vi "Read Multi Digital.vi"(0 "Device ID":T3(ring), 5 "Module":T2(array[ring]), 7 "Digital Input":T1(array[ring]), 11 "error in":errorcluster) -> (4 "Device ID Out":T3(ring), 6 "Value":bool[](array[boolean]), 15 "error out":errorcluster)   [LabVIEW 2010]
doc: "This VI reads multiple digital inputs from the transfer area."
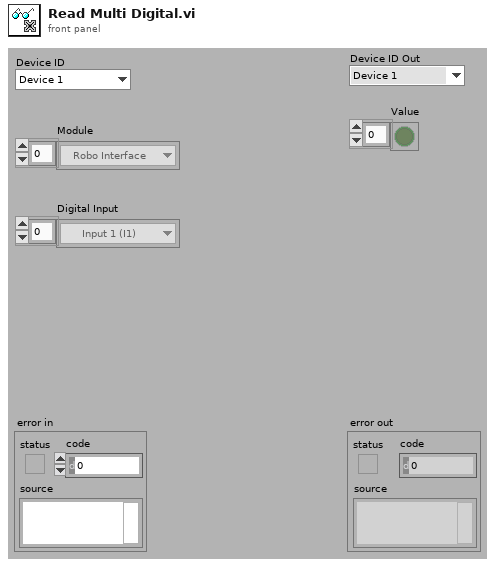
[diagram p1: front panel]
types:
  T1 = enum8{"Input 1 (I1)", "Input 2 (I2)", "Input 3 (I3)", "Input 4 (I4)", "Input 5 (I5)", "Input 6 (I6)", "Input 7 (I7)", "Input 8 (I8)"}[]
  T2 = enum8{"Robo Interface", "Extension 1", "Extension 2", "Extension 3"}[]
  T3 = enum16{"Device 1", "Device 2", "Device 3", "Device 4", "Device 5", "Device 6", "Device 7", "Device 8"}
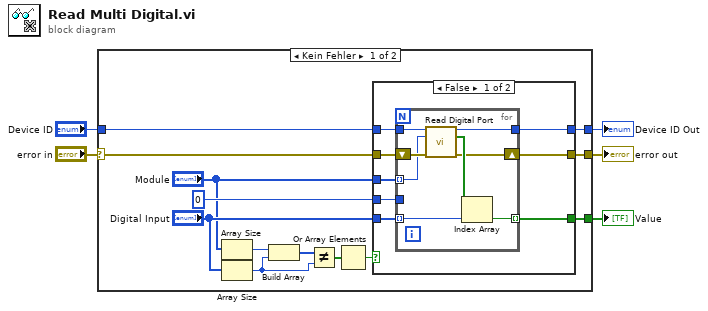
[diagram p0: block diagram]
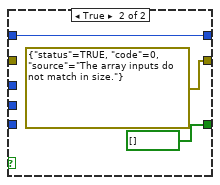
[diagram p2: hidden frame]
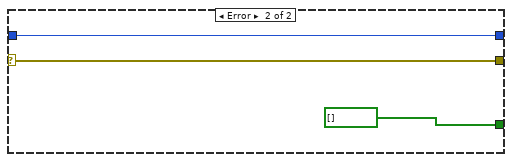
[diagram p3: hidden frame]
diagram:
  n1 = case shown="Kein Fehler" "error in" {
    selector: "error in" -> [w16 w40]
    tunnel: [w15 w40] -> w4
    tunnel: "Device ID" -> [w7 w39]
    tunnel: [w6 w39] -> w2
    tunnel: [w17 bool[] []] -> w1
    frame No Error {
      n2 = Array Size(array="Module") -> (size(s)=w14:i32)
      n3 = Array Size(array="Digital Input") -> (size(s)=w12:i32)
      n4 = Build Array(w14, w12) -> (w13:i32[])
      n5 = Not Equal?(x=w13, y=w12) -> (x != y?=w11:bool[])
      n6 = Or Array Elements(Boolean array=w11) -> (logical OR=w9:bool)
      n7 = case shown="FALSE" w9 {
        tunnel: u8 0 ("unsigned 8bit integer") -> [w26 _]
        tunnel: "Module" -> [w25 _]
        tunnel: [w24 bool[] []] -> w17
        tunnel: w16 -> [w23 _]
        tunnel: w7 -> [w22 w35]
        tunnel: [w21 errorcluster {"status"=TRUE, "code"=0, "source"="The array inputs do not match in size."} ("error out")] -> w15
        tunnel: "Digital Input" -> [w20 _]
        tunnel: [w19 w35] -> w6
        frame False {
          n8 = for {
            tunnel: w26 -> [_]
            tunnel: w25 -> [w28] mode=indexing
            tunnel: w20 -> [w34] mode=indexing
            tunnel: [w33] -> w24 mode=indexing
            shift-right: [w30] -> w21
            shift-left: w23 -> [w32]
            tunnel: w22 -> [w29]
            tunnel: [w27] -> w19
            n9 = call "Read Digital Port.vi"("Device ID"=w29, "Module"=w28, "error in"=w32) -> ("Device ID Out"=w27:T3, "Value"=w31:bool[], "error out"=w30:errorcluster)  [unwired: 10 out]
            n10 = Index Array(array=w31, index=w34) -> (element=w33:bool)
          }
        }
        frame True {
        }
      }
    }
    frame Error {
    }
  }
  "error out" <- w4
  "Device ID Out" <- w2
  "Value" <- w1
